vi "RotateHWP.vi"(6 "Action":T1=enum."Get Moving", 8 "error in":errorcluster, 9 "Set Angle":u32 max=355 step=5, 11 "VISA Refnum in":refnum<visa-resource-name>="COM1") -> (0 "error out":errorcluster, 2 "Read Buffer":string, 3 "VISA resource name out":refnum<visa-resource-name>)   [LabVIEW 2014]
doc: "Connects and Disconnects theserial port to the HWP.\nRotates the Half-Wave Plate to a Set Angle. \nZeros the HWP - rotate to zero degrees. \nCalibrates the HWP - rotates the HWP by 360 degrees and averages the time taken between 35 ten degree interrupts. Half of this is set to the time taken to rotate by 5 degrees.\nGets whether the HWP is rotating currently.\nGets the current angle that the HWP is at currently."
uses:
  RotateHWP.ctl
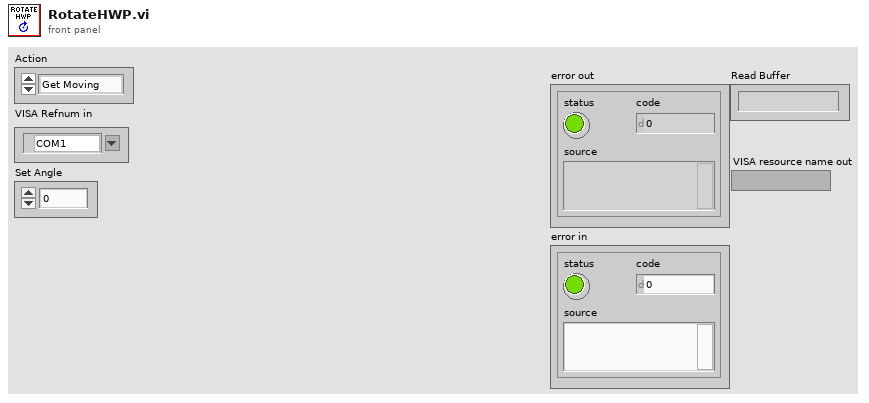
[diagram p1: front panel]
types:
  T1 = typedef "RotateHWP.ctl" = enum16{"Connect", "Disconnect", "Get Moving", "Set Zero", "Set Angle", "Get Angle", "Calibrate"}
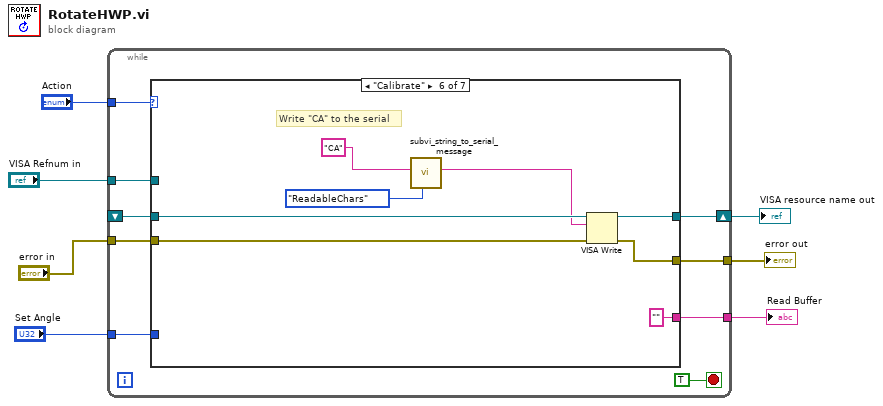
[diagram p0: block diagram]
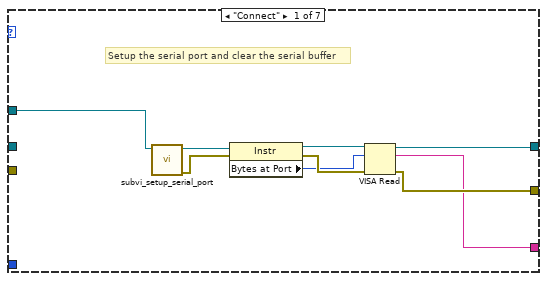
[diagram p2: hidden frame]
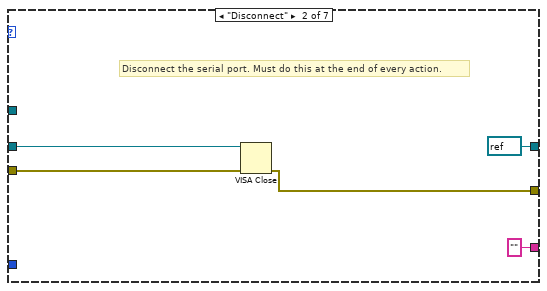
[diagram p3: hidden frame]
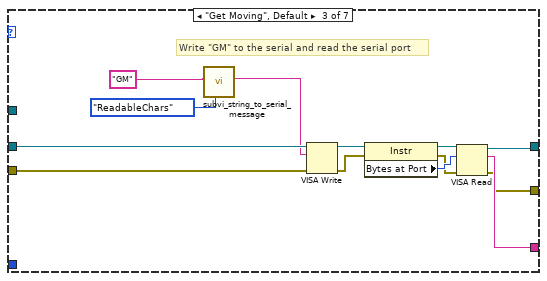
[diagram p4: hidden frame]
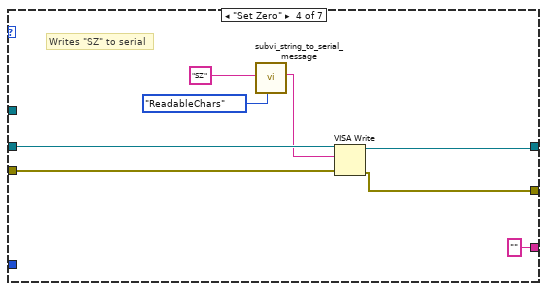
[diagram p5: hidden frame]
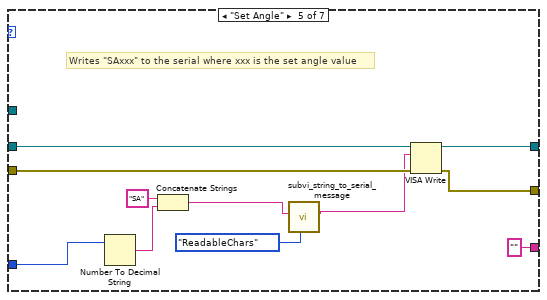
[diagram p6: hidden frame]
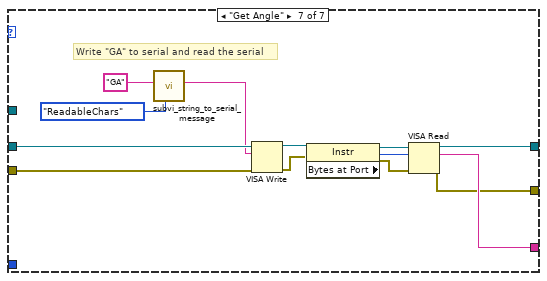
[diagram p7: hidden frame]
diagram:
  n1 = while {
    tunnel: "Action" -> [w16]
    tunnel: [w14] -> w5
    shift-right: [w15] -> w6
    shift-left: _ -> [w13]
    tunnel: "error in" -> [w11]
    tunnel: [w10] -> w3
    tunnel: "Set Angle" -> [w9]
    tunnel: "VISA Refnum in" -> [w8]
    stop <- TRUE stop-if-true
    n2 = case shown="\"Calibrate\"" w16 {
      tunnel: [w20 refnum<visa-resource-name> refnum ("VISA Refnum out") w35 w49 w57 w69 w82] -> w15
      tunnel: [w19 w28 w34 w48 w56 w68 w81] -> w14
      tunnel: w13 -> [_ w30 w43 w51 w59 w67 w76]
      tunnel: w11 -> [_ w29 w42 w50 w58 w66 w75]
      tunnel: [w18 "" ("read buffer") w36 "" ("read buffer") "" ("read buffer") "" ("read buffer") w83] -> w10
      tunnel: w9 -> [_ _ _ _ w61 _ _]
      tunnel: w8 -> [w17 _ _ _ _ _ _]
      frame "Connect" {
        # "Setup the serial port and clear the serial buffer"
        n3 = call "subvi_setup_serial_port.vi"("VISA Refnum in"=w17) -> ("error out"=w24:errorcluster, "VISA Refnum out"=w25:refnum<visa-resource-name>)  [unwired: 9 in]
        n4 = property class="Instr"(reference=w25, error in=w24) -> (reference out=w23:refnum<visa-resource-name>, error out=w22:errorcluster, "Bytes at Port"=w21:u32)
        n5 = VISA Read(VISA resource name=w23, byte count=w21, error in (no error)=w22) -> (VISA resource name out=w20:refnum<visa-resource-name>, read buffer=w18:string, error out=w19:errorcluster)  [unwired: 1 out]
      }
      frame "Disconnect" {
        # "Disconnect the serial port. Must do this at the end of every action."
        n6 = VISA Close(VISA resource name=w30, error in (no error)=w29) -> (error out=w28:errorcluster)
      }
      frame "Get Moving", Default {
        # "Write \"GM\" to the serial and read the serial port"
        n7 = call "subvi_string_to_serial_message.vi"("Type"=enum16{"ReadableChars", "SpellmanMPS"}."ReadableChars", "Input Message"="GM" ("write buffer")) -> ("Serial Message"=w32:string)  [unwired: 9 in]
        n8 = VISA Write(VISA resource name=w43, write buffer=w32, error in (no error)=w42) -> (VISA resource name out=w41:refnum<visa-resource-name>, error out=w40:errorcluster)  [unwired: 1 out]
        n9 = property class="Instr"(reference=w41, error in=w40) -> (reference out=w38:refnum<visa-resource-name>, error out=w37:errorcluster, "Bytes at Port"=w39:u32)
        n10 = VISA Read(VISA resource name=w38, byte count=w39, error in (no error)=w37) -> (VISA resource name out=w35:refnum<visa-resource-name>, read buffer=w36:string, error out=w34:errorcluster)  [unwired: 1 out]
      }
      frame "Set Zero" {
        # "Writes \"SZ\" to serial"
        n11 = call "subvi_string_to_serial_message.vi"("Type"=enum16{"ReadableChars", "SpellmanMPS"}."ReadableChars", "Input Message"="SZ" ("write buffer")) -> ("Serial Message"=w45:string)  [unwired: 9 in]
        n12 = VISA Write(VISA resource name=w51, write buffer=w45, error in (no error)=w50) -> (VISA resource name out=w49:refnum<visa-resource-name>, error out=w48:errorcluster)  [unwired: 1 out]
      }
      frame "Set Angle" {
        # "Writes \"SAxxx\" to the serial where xxx is the set angle value"
        n13 = Number To Decimal String(number=w61) -> (decimal integer string=w60:string)  [unwired: 1 in]
        n14 = Concatenate Strings("SA" ("string"), w60) -> (w54:string)
        n15 = call "subvi_string_to_serial_message.vi"("Type"=enum16{"ReadableChars", "SpellmanMPS"}."ReadableChars", "Input Message"=w54) -> ("Serial Message"=w53:string)  [unwired: 9 in]
        n16 = VISA Write(VISA resource name=w59, write buffer=w53, error in (no error)=w58) -> (VISA resource name out=w57:refnum<visa-resource-name>, error out=w56:errorcluster)  [unwired: 1 out]
      }
      frame "Calibrate" {
        # "Write \"CA\" to the serial"
        n17 = call "subvi_string_to_serial_message.vi"("Type"=enum16{"ReadableChars", "SpellmanMPS"}."ReadableChars", "Input Message"="CA") -> ("Serial Message"=w64:string)  [unwired: 9 in]
        n18 = VISA Write(VISA resource name=w67, write buffer=w64, error in (no error)=w66) -> (VISA resource name out=w69:refnum<visa-resource-name>, error out=w68:errorcluster)  [unwired: 1 out]
      }
      frame "Get Angle" {
        # "Write \"GA\" to serial and read the serial"
        n19 = call "subvi_string_to_serial_message.vi"("Type"=enum16{"ReadableChars", "SpellmanMPS"}."ReadableChars", "Input Message"="GA" ("write buffer")) -> ("Serial Message"=w72:string)  [unwired: 9 in]
        n20 = VISA Write(VISA resource name=w76, write buffer=w72, error in (no error)=w75) -> (VISA resource name out=w80:refnum<visa-resource-name>, error out=w74:errorcluster)  [unwired: 1 out]
        n21 = property class="Instr"(reference=w80, error in=w74) -> (reference out=w78:refnum<visa-resource-name>, error out=w77:errorcluster, "Bytes at Port"=w79:u32)
        n22 = VISA Read(VISA resource name=w78, byte count=w79, error in (no error)=w77) -> (VISA resource name out=w82:refnum<visa-resource-name>, read buffer=w83:string, error out=w81:errorcluster)  [unwired: 1 out]
      }
    }
  }
  "error out" <- w5
  "VISA resource name out" <- w6
  "Read Buffer" <- w3
